vi "MAIN.vi"() -> ()   [LabVIEW 2011]
doc: "Use this template to build a standard state machine design pattern. Each state executes code and determines which state to transition to. Contrast this design pattern with the User Interface Event Handler pattern, in which code executes in response to user actions. Contrast this design pattern also with the Queued Message Handler pattern, in which each message handling code can queue zero or more new messages."
uses:
  SubVI/Control/Status.ctl
  SubVI/Global.vi
panel:
  out "String":string
  in  "Settings Button":bool
  out "match?":bool
  out "match?":bool
  out "SN2":string
  out "SN1":string
  out "Status":T1
  in  "Cancel Button":bool
  in  "OK Button":bool
  # "Provided by KSHJT@2018"
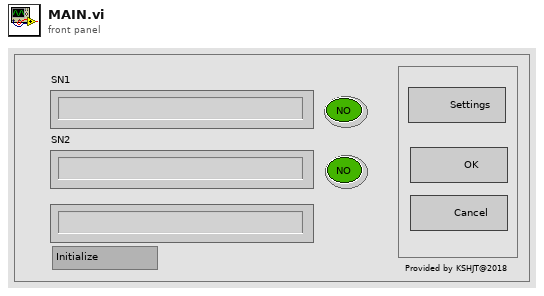
[diagram p1: front panel]
types:
  T1 = typedef "Status.ctl" = enum16{"Initialize", "IDLE", "Scan", "SN_Check", "MonitorResult", "Report", "Stop"}
  T2 = cluster{"Label1":string, "Label2":string, "Test_Time":string, "Model_Name":string, "Test_Result":string}
  T3 = cluster{"Fix_SN2":string, "Offset_SN2":u32, "Fix_SN2_Length":u32}
  T4 = cluster{"Fix_SN1":string, "Offset_SN1":u32, "Fix_SN1_Length":u32}
  T5 = cluster{"Label1":string, "Label2":string, "Model_Name":string, "Test_Time":string, "Test_Result":string, "DSN":string, "Table_Name":string}
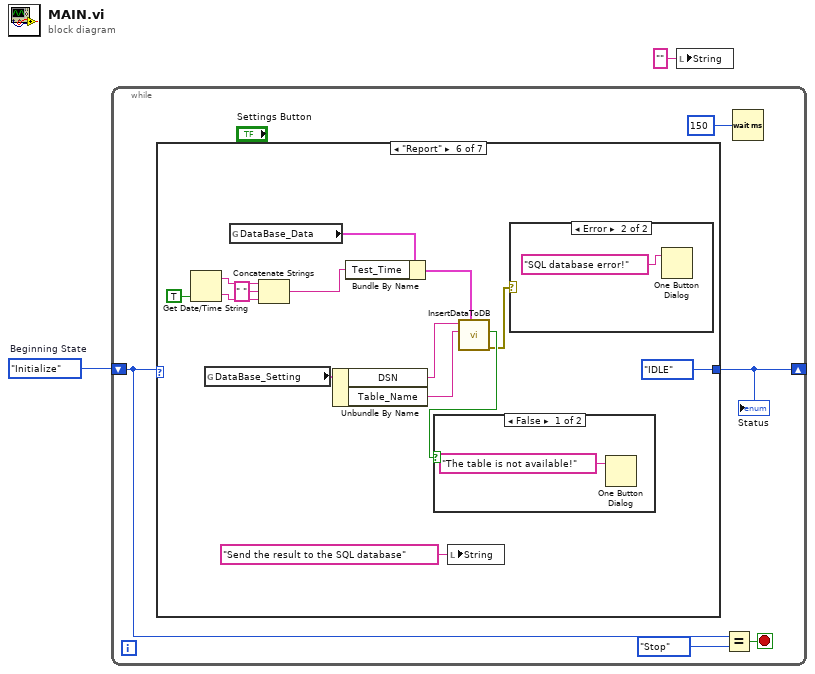
[diagram p0: block diagram]
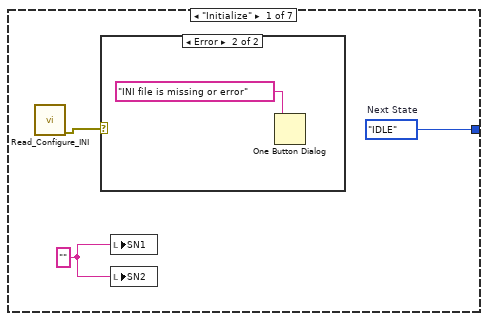
[diagram p2: hidden frame]
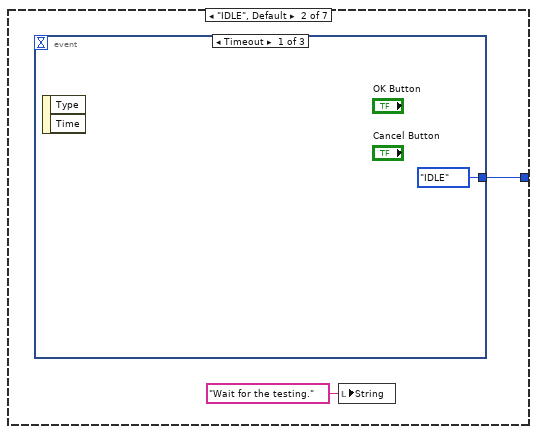
[diagram p4: hidden frame]
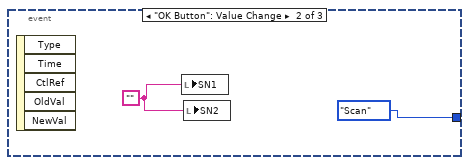
[diagram p5: hidden frame]
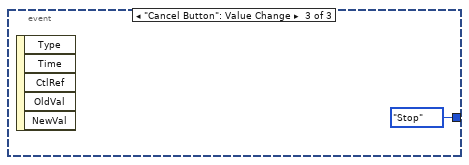
[diagram p6: hidden frame]
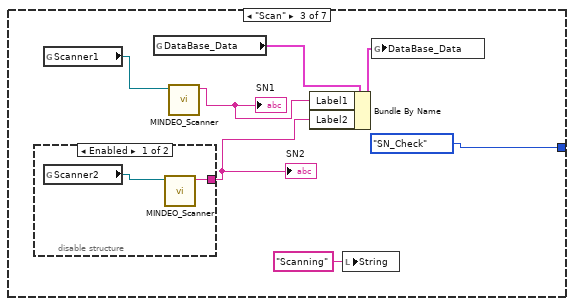
[diagram p7: hidden frame]
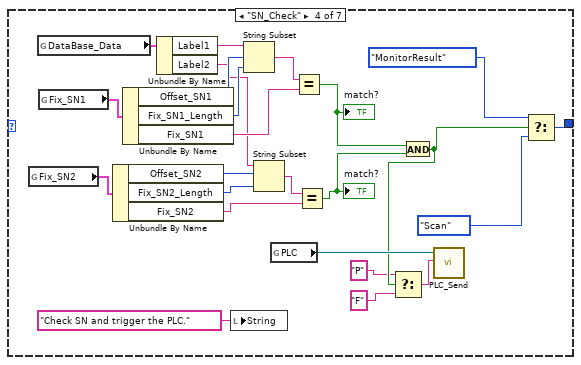
[diagram p9: hidden frame]
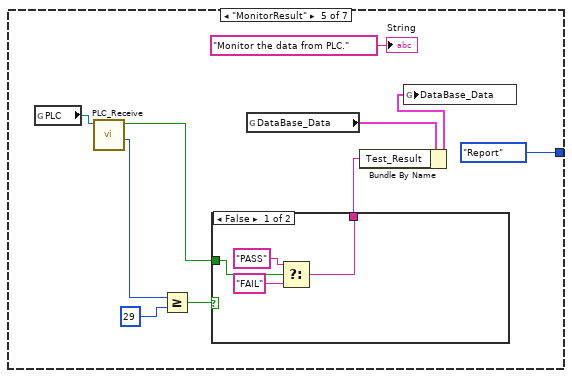
[diagram p10: hidden frame]
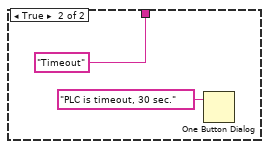
[diagram p11: hidden frame]
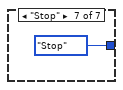
[diagram p14: hidden frame]
diagram:
  w2 = Status."Initialize"  # Beginning State
  n1 = while {
    shift-right: [w4] -> _
    shift-left: w2 -> [w5]
    stop <- w7 stop-if-true
    n2 = case shown="\"Report\"" w5 {
      tunnel: [w10 w13 Status."SN_Check" ("Next State") w49 Status."Report" ("Next State") Status."IDLE" ("Next State") Status."Stop" ("Next State")] -> w4
      frame "Initialize" {
        w8 = ""
        w10 = Status."IDLE"  # Next State
        n3 = call "Read_Configure_INI.vi"() -> ("error out"=w9:errorcluster)  [unwired: 11 in]
        n4 = case shown="Error" w9 {
          frame No Error {
          }
          frame Error {
            n5 = One Button Dialog(message="INI file is missing or error") -> ()  [unwired: 1 in, 1 out]
          }
        }
        n6 = local write "SN1"(w8) -> ()
        n7 = local write "SN2"(w8) -> ()
      }
      frame "IDLE", Default {
        n8 = event shown="[0] Timeout" {
          selector: _ -> [_ _ _]
          dyn-events: _ -> [_ _ _]
          timeout: _ -> [_ _ _]
          tunnel: [Status."IDLE" ("Next State") Status."Scan" ("Next State") Status."Stop" ("Next State")] -> w13
          event Timeout {
            n9 = event-data() -> ()  [unwired: 1 in, 2 out]
          }
          event "OK Button": Value Change {
            w15 = ""
            n10 = event-data() -> ()  [unwired: 1 in, 5 out]
            n11 = local write "SN1"(w15) -> ()
            n12 = local write "SN2"(w15) -> ()
          }
          event "Cancel Button": Value Change {
            n13 = event-data() -> ()  [unwired: 1 in, 5 out]
          }
        }
        n14 = local write "String"("Wait for the testing." ("String")) -> ()
      }
      frame "Scan" {
        n15 = disable-structure shown="Enabled" {
          disable-tunnel: [w25 _] -> w18
          frame Enabled {
            n16 = global read "Global.vi" "Scanner2"() -> (w26:refnum<visa-resource-name>)
            n17 = call "MINDEO_Scanner.vi"("VISA resource name"=w26) -> ("trimmed string"=w25:string)  [unwired: 9 in, 1 out]
          }
          frame Disabled {
          }
        }
        "SN2" <- w18
        n18 = global read "Global.vi" "Scanner1"() -> (w23:refnum<visa-resource-name>)
        n19 = global read "Global.vi" "DataBase_Data"() -> (w21:T2)
        n20 = call "MINDEO_Scanner.vi"("VISA resource name"=w23) -> ("trimmed string"=w20:string)  [unwired: 9 in, 1 out]
        "SN1" <- w20
        n21 = Bundle By Name(cluster=w21, "Label1"=w20, "Label2"=w18) -> (w22:T2)
        n22 = local write "String"("Scanning" ("String")) -> ()
        n23 = global write "Global.vi" "DataBase_Data"(w22) -> ()
      }
      frame "SN_Check" {
        n24 = global read "Global.vi" "Fix_SN2"() -> (w40:T3)
        n25 = global read "Global.vi" "DataBase_Data"() -> (w47:T2)
        n26 = global read "Global.vi" "Fix_SN1"() -> (w45:T4)
        n27 = Unbundle By Name(w40) -> ("Offset_SN2"=w39:u32, "Fix_SN2_Length"=w37:u32, "Fix_SN2"=w35:string)
        n28 = Unbundle By Name(w45) -> ("Offset_SN1"=w44:u32, "Fix_SN1_Length"=w43:u32, "Fix_SN1"=w41:string)
        n29 = Unbundle By Name(w47) -> ("Label1"=w46:string, "Label2"=w38:string)
        n30 = local write "String"("Check SN and trigger the PLC." ("String")) -> ()
        n31 = String Subset(string=w46, offset (0)=w44, length (rest)=w43) -> (substring=w42:string)
        n32 = String Subset(string=w38, offset (0)=w39, length (rest)=w37) -> (substring=w36:string)
        n33 = global read "Global.vi" "PLC"() -> (w32:refnum<visa-resource-name>)
        n34 = Equal?(x=w42, y=w41) -> (x = y?=w34:bool)
        "match?" <- w34
        n35 = Equal?(x=w36, y=w35) -> (x = y?=w33:bool)
        "match?" <- w33
        n36 = And(x=w34, y=w33) -> (x .and. y?=w31:bool)
        n37 = Select(t="P", s=w31, f="F") -> (s? t:f=w29:string)
        n38 = call "PLC_Send.vi"("P/F"=w29, "VISA resource name"=w32) -> ()  [unwired: 9 in, 1 out]
        n39 = Select(t=Status."MonitorResult" ("Next State"), s=w31, f=Status."Scan" ("Next State")) -> (s? t:f=w49:T1)
      }
      frame "MonitorResult" {
        n40 = global read "Global.vi" "PLC"() -> (w58:refnum<visa-resource-name>)
        n41 = call "PLC_Receive.vi"("VISA resource name"=w58) -> ("loops(29)"=w56:i32, "pass?"=w52:bool)  [unwired: 7 in, 2 out]
        n42 = Greater Or Equal?(x=w56, y=29) -> (x >= y?=w54:bool)
        n43 = case shown="False" w54 {
          tunnel: w52 -> [w64 _]
          tunnel: [w62 "Timeout"] -> w51
          frame False {
            n44 = Select(t="PASS", s=w64, f="FAIL") -> (s? t:f=w62:string)
          }
          frame True {
            n45 = One Button Dialog(message="PLC is timeout, 30 sec.") -> ()  [unwired: 1 in, 1 out]
          }
        }
        n46 = global read "Global.vi" "DataBase_Data"() -> (w60:T2)
        n47 = Bundle By Name(cluster=w60, "Test_Result"=w51) -> (w59:T2)
        n48 = global write "Global.vi" "DataBase_Data"(w59) -> ()
        "String" <- "Monitor the data from PLC." ("String")
      }
      frame "Report" {
        n49 = Get Date/Time String(want seconds? (F)=TRUE) -> (date string=w72:string, time string=w71:string)  [unwired: 2 in]
        n50 = global read "Global.vi" "DataBase_Setting"() -> (w79:T5)
        n51 = global read "Global.vi" "DataBase_Data"() -> (w74:T2)
        n52 = Concatenate Strings(w72, " " ("string"), w71) -> (w68:string)
        n53 = Unbundle By Name(w79) -> ("DSN"=w78:string, "Table_Name"=w77:string)
        n54 = Bundle By Name(cluster=w74, "Test_Time"=w68) -> (w73:T2)
        n55 = local write "String"("Send the result to the SQL database" ("String")) -> ()
        n56 = call "InsertDataToDB.vi"("data"=w73, "table"=w77, "DSN"=w78) -> ("error out"=w75:errorcluster, "table?"=w76:bool)  [unwired: 6 in, 1 out]
        n57 = case shown="False" w76 {
          frame False {
            n58 = One Button Dialog(message="The table is not available!") -> ()  [unwired: 1 in, 1 out]
          }
          frame True {
          }
        }
        n59 = case shown="Error" w75 {
          frame No Error {
          }
          frame Error {
            n60 = One Button Dialog(message="SQL database error!") -> ()  [unwired: 1 in, 1 out]
          }
        }
      }
      frame "Stop" {
      }
    }
    "Status" <- w4
    n61 = Equal?(x=w5, y=Status."Stop" ("States")) -> (x = y?=w7:bool)
    n62 = Wait (ms)(milliseconds to wait=u32 150) -> ()  [unwired: 1 out]
  }
  n63 = local write "String"("" ("String")) -> ()
